vi "Subvi AO mon.vi"(1 "AO mon":refnum<k21>="Connector1/AO1", 2 "AO":refnum<k21>="Connector1/AO0", 7 "Ext trig enable":bool, 9 "FIFO In":refnum<k21>="AB0") -> ()   [LabVIEW 2017]
uses:
  <vilib>/rvi/Emulation/niFpgaGetClockAttributes.vi
  <vilib>/rvi/Emulation/niFpgaSctlEmulationGetInTimedLoop.vi
  <vilib>/rvi/Emulation/niFpgaEmulationReportErrorSimple.vi
  Detector/GV frameclock.vi
  <vilib>/rvi/Emulation/niFpgaCriticalErrorInLSC.vi
  GV FIFO timeout.vi
  <vilib>/rvi/eio/common/nirviEmuTemplateMethod_errors.vi
  <vilib>/rvi/DataTransferAndStorage/Container/Common/niFpgaContainerExecOnDevCompGetState.vi
  <vilib>/rvi/Emulation/niFpgaEmulationIsFPGAContextNoSignature.vi
  <vilib>/rvi/errors/niFpgaSetErrorForExecOnDevCompSimple.vi
  <vilib>/rvi/eio/common/nirviEmuReportErrorAndStop.vi
  <vilib>/rvi/DataTransferAndStorage/Container/Common/niFpgaContainerGetUniqueNameForEmu.vi
  <vilib>/rvi/FIFO/Fifo_Resource/nirvififoEmulationSetSize.vi
  <vilib>/rvi/FIFO/Fifo_Resource/nirviFifoEmulationQueueMgr.vi
  <instcachedir>/0/nirviFifoEmulationQueueMgr_E5CAEC123FF24DC58D834DCA3CDAA9B5.lvgen/nirviFifoEmulationQueueMgr_E5CAEC123FF24DC58D834DCA3CDAA9B5_001.vi
  <vilib>/rvi/FIFO/Fifo_Resource/nirvififoEmulationDetermineInputValidOut.vi
  <vilib>/rvi/FIFO/Fifo_Resource/nirvififoEmulationCreateLock.vi
  <vilib>/rvi/Emulation/niFpgaProcessEmulError.vi
  <vilib>/rvi/FIFO/Fifo_Resource/nirvififoEmulationObtainLock.vi
  <vilib>/rvi/FIFO/Fifo_Resource/nirvififoEmulationReleaseLock.vi
  <vilib>/rvi/occurrence/nirviWaitOnOccurrenceBase.vi
  <vilib>/rvi/errors/nirviReportUnexpectedCaseInternalError.vi
  <vilib>/rvi/errors/nirviReportUnexpectedCaseInternalError (U32).vi
  <vilib>/Utility/error.llb/Clear Errors.vi
  <vilib>/rvi/interface/RandomDataEmulation/niFpgaRandomDataHandleErrors.vi
  <vilib>/eio/EIONode/EIONode.xnode
  <vilib>/rvi/DataTransferAndStorage/Container/XNode/niFpgaContainer.xnode
  <vilib>/rvi/FIFO/Fifo_Resource/niFpgaFifoEmulationRefIn.vi
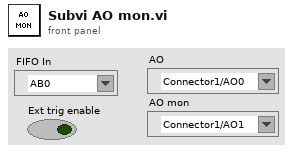
[diagram p1: front panel]
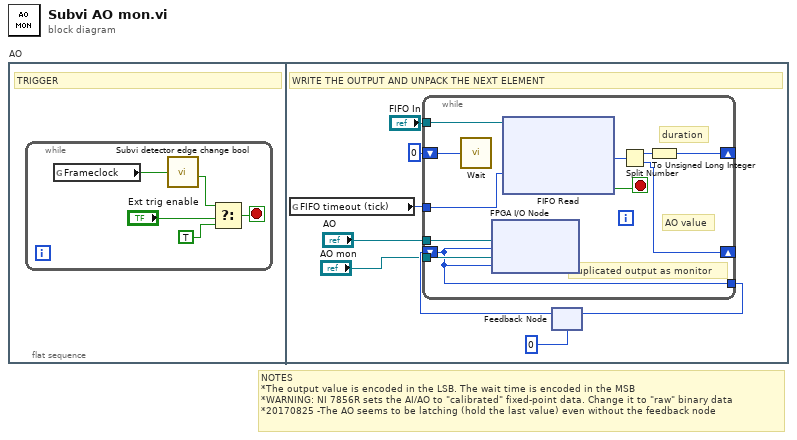
[diagram p0: block diagram]
diagram:
  # "NOTES\n*The output value is encoded in the LSB. The wait time is encoded in the MSB\n*WARNING: NI 7856R sets the AI/AO to \"calibrated\" fixed-point data. Change it to \"raw\" binary data\n*20170825 -The AO seems to be latching (hold the last value) even without the feedback node"
  n1 = flat-sequence "AO" {
    frame #0 {
      # "TRIGGER"
      n2 = while {
        stop <- w2 stop-if-true
        n3 = global read "GV frameclock.vi" "Frameclock"() -> (w5:bool)
        n4 = call "Subvi detector edge change bool.vi"("Input"=w5) -> ("Output"=w1:bool)  [unwired: 8 in]
        n5 = Select(t=w1, s="Ext trig enable", f=TRUE) -> (s? t:f=w2:bool)
      }
    }
    frame #1 {
      # "WRITE THE OUTPUT AND UNPACK THE NEXT ELEMENT"
      n6 = global read "GV FIFO timeout.vi" "FIFO timeout (tick)"() -> (w9:i32)
      n7 = feedback #1(u16 0) -> (w12:u16)
      n8 = while {
        shift-right: [w17] -> _
        shift-left: u32 0 -> [w24]
        shift-right: [w22] -> _
        shift-left: w12 -> [w14]
        tunnel: [w14] -> w10
        tunnel: "FIFO In" -> [w19]
        tunnel: w9 -> [w18]
        tunnel: "AO" -> [w16]
        tunnel: "AO mon" -> [w15]
        stop <- w20 stop-if-true
        # "duplicated output as monitor"
        # "duration"
        # "AO value"
        n9 = call "Wait"("Count(Ticks)"=w24) -> ()  [unwired: 1 out]
        n10 = xnode "FPGA I/O Node"("I/O Item"=w14, "FPGA I/O In"=w16, "I/O Item"=w14, "FPGA I/O In"=w15) -> ()  [unwired: 2 out]
        n11 = xnode ("FIFO Read")("Timeout"=w18, "FIFO In"=w19) -> ("Element"=w21:u32, "Timed Out?"=w20:bool)  [unwired: 1 out]
        n12 = Split Number(x=w21) -> (hi(x)=w23:u16, lo(x)=w22:u16)
        n13 = To Unsigned Long Integer(number=w23) -> (unsigned 32bit integer=w17:u32)
      }
      n14 = feedback-in #1(w10) -> ()
    }
  }
